vi "ATF-Pump-ACC_Scale.vi"(8 "error in (no error)":errorcluster, 10 "Accelerometer":T1(array[cluster]), 11 "Refnum in":refnum<k21>) -> (0 "error out":errorcluster, 3 "Refnum out":refnum<k21>)   [LabVIEW 2022 SP3]
uses:
  <vilib>/DAQmx/create/channels.llb/DAQmx Create Channel (AI-Acceleration-Accelerometer).vi
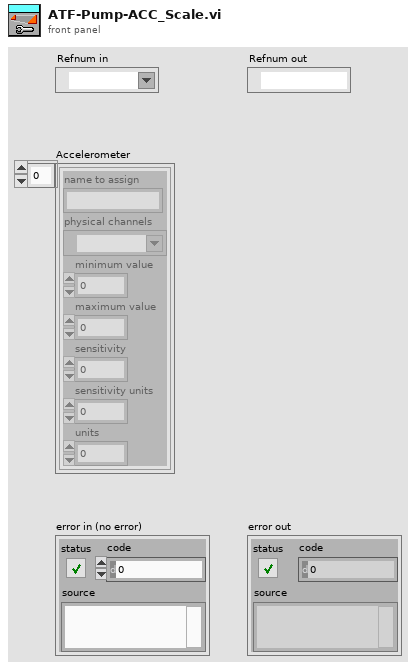
[diagram p1: front panel]
types:
  T1 = cluster{"name to assign":string, "physical channels":tag, "minimum value":dbl, "maximum value":dbl, "sensitivity":dbl, "sensitivity units":i32, "units":i32}[]
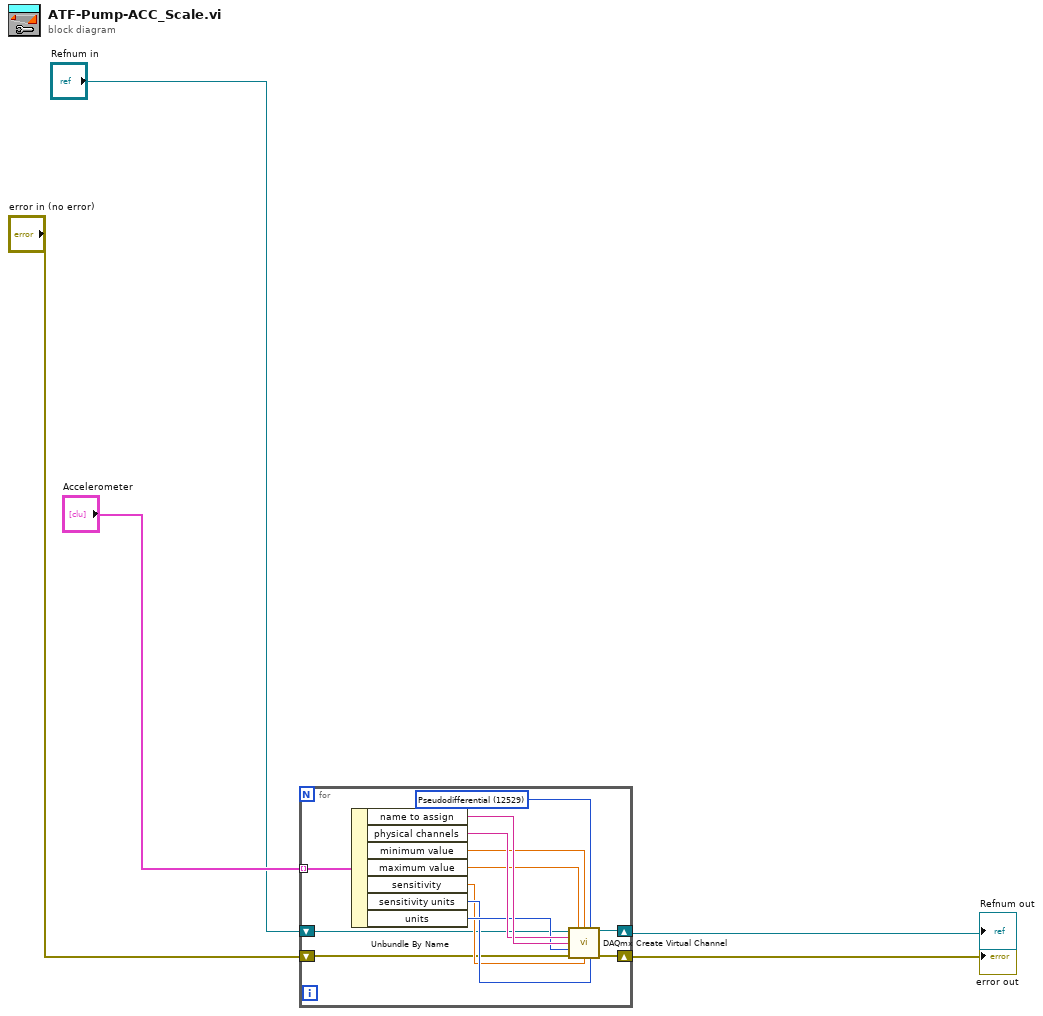
[diagram p0: block diagram]
diagram:
  n1 = for {
    tunnel: "Accelerometer" -> [w18] mode=indexing
    shift-right: [w9] -> w1
    shift-left: "error in (no error)" -> [w8]
    shift-right: [w10] -> w2
    shift-left: "Refnum in" -> [w6]
    w7 = 12529 items=["default"=-1, "RSE"=10083, "NRSE"=10078, "Differential"=10106, "Pseudodifferential"=12529] ("input terminal configuration")
    n2 = Unbundle By Name(w18) -> ("name to assign"=w17:string, "physical channels"=w16:tag, "minimum value"=w12:dbl, "maximum value"=w11:dbl, "sensitivity"=w13:dbl, "sensitivity units"=w14:i32, "units"=w15:i32)
    n3 = call-poly <vilib>:"DAQmx Create Virtual Channel.vi"("task in"=w6, "maximum value"=w11, "minimum value"=w12, "input terminal configuration"=w7, "physical channels"=w16, "name to assign"=w17, "units"=w15, "error in"=w8, "sensitivity"=w13, "sensitivity units"=w14) -> ("task out"=w10:refnum<k21>, "error out"=w9:errorcluster)  [unwired: 4 in]
  }
  "Refnum out" <- w2
  "error out" <- w1
